vi "Create RND Path.vi"(11 "Coordinate[] In":T1[](array[typedef])=[{"x"=67.57906304229073, "y"=68.60831518225434}, {"x"=81.83522625397705, "y"=7.983158550148239}, {"x"=13.845000200345314, "y"=50.20462870854803}, {"x"=65.60632392598347, "y"=23.41592963463568}, {"x"=37.527186631799125, "y"=49.26560940206024}, {"x"=75.80408834272797, "y"=82.83507884873025}, {"x"=91.24590880296392, "y"=43.00621931342281}, {"x"=88.66715419959786, "y"=61.38804665807669}, {"x"=86.51526432096372, "y"=8.714647141634234}, {"x"=83.91892871742184, "y"=30.341190073224354}, {"x"=24.743038312024, "y"=79.88068424696041}, {"x"=25.30168704115323, "y"=47.03932115592622}, {"x"=88.22800157317587, "y"=11.43101038338128}]) -> (3 "Coordinate[] Out":T1[](array[typedef])=[{"x"=67.57906304229073, "y"=68.60831518225434}, {"x"=81.83522625397705, "y"=7.983158550148239}, {"x"=13.845000200345314, "y"=50.20462870854803}, {"x"=65.60632392598347, "y"=23.41592963463568}, {"x"=37.527186631799125, "y"=49.26560940206024}, {"x"=75.80408834272797, "y"=82.83507884873025}, {"x"=91.24590880296392, "y"=43.00621931342281}, {"x"=88.66715419959786, "y"=61.38804665807669}, {"x"=86.51526432096372, "y"=8.714647141634234}, {"x"=83.91892871742184, "y"=30.341190073224354}, {"x"=24.743038312024, "y"=79.88068424696041}, {"x"=25.30168704115323, "y"=47.03932115592622}, {"x"=88.22800157317587, "y"=11.43101038338128}])   [LabVIEW 2015, in "TSP Library.lvlib"]
uses:
  TSP Library.lvlib
  TypeDef/Coordinate.ctl
  <vilib>/Analysis/NI_AALBase.lvlib
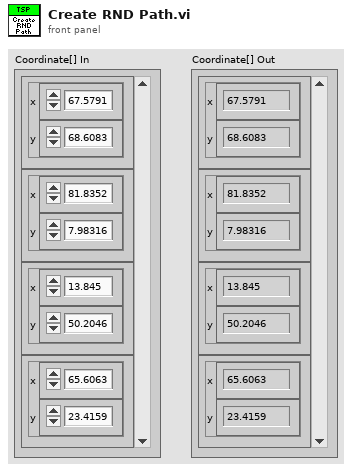
[diagram p1: front panel]
types:
  T1 = typedef "TSP Library.lvlib/Coordinate.ctl" = cluster{"x":dbl, "y":dbl}
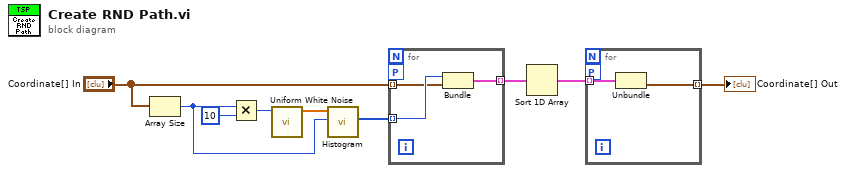
[diagram p0: block diagram]
diagram:
  n1 = Array Size(array="Coordinate[] In") -> (size(s)=w6:i32)
  n2 = Multiply(x=w6, y=10) -> (x*y=w8:i32)
  n3 = call <vilib>:"Uniform White Noise.vi"("samples"=w8) -> ("uniform white noise"=w7:dbl[])  [unwired: 9 in, 1 out]
  n4 = call <vilib>:"Histogram.vi"("intervals"=w6, "X"=w7) -> ("Histogram: h(x)"=w4:i32[])  [unwired: 6 in, 3 out]
  n5 = for {
    tunnel: "Coordinate[] In" -> [w11] mode=indexing
    tunnel: w4 -> [w12] mode=indexing
    tunnel: [w10] -> w3 mode=indexing
    workers-P: _ -> [_]
    n6 = Bundle(w12, "Coordinate"=w11) -> (w10:cluster{i32, "Coordinate":T1})  [unwired: 1 in]
  }
  n7 = Sort 1D Array(array=w3) -> (sorted array=w2:cluster{i32, "Coordinate":T1}[])
  n8 = for {
    tunnel: w2 -> [w14] mode=indexing
    tunnel: [w13] -> w1 mode=indexing
    workers-P: _ -> [_]
    n9 = Unbundle(w14) -> ("Coordinate"=w13:T1)  [unwired: 1 out]
  }
  "Coordinate[] Out" <- w1
